vi "Error Handler - UI Loop - cRIO Target Monitoring.vi"(8 "error in (no error)":errorcluster caption="错误输入（无错误）", 11 "Message Queue":refnum<queue> caption="消息队列") -> (3 "dup Message Queue":refnum<queue> caption="消息队列副本")   [LabVIEW 2015]
uses:
  Support VIs/Message Queue/Message Cluster.ctl
  Support VIs/Message Queue/Message Queue.lvlib
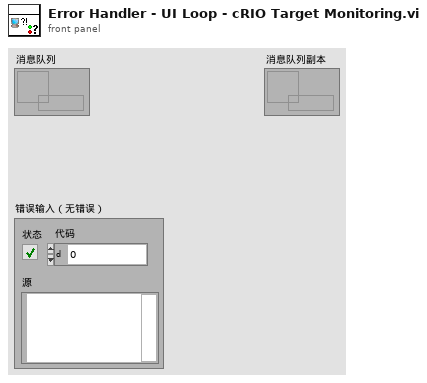
[diagram p1: front panel]
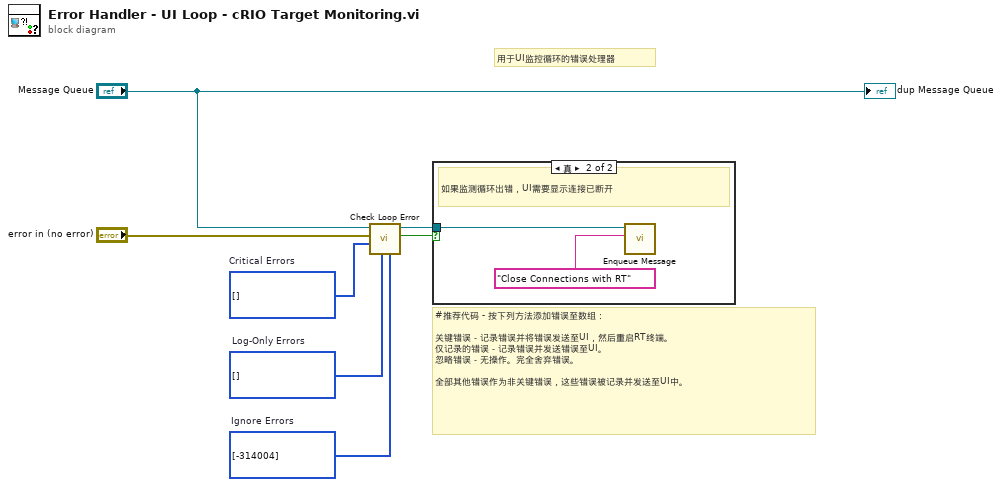
[diagram p0: block diagram]
diagram:
  w5 = i32[] [-314004]  # Ignore Errors
  w6 = i32[] []  # Log-Only Errors
  w7 = i32[] []  # Critical Errors
  # "#推荐代码 - 按下列方法添加错误至数组：\n\n关键错误－记录错误并将错误发送至UI，然后重启RT终端。\n仅记录的错误－记录错误并发送错误至UI。\n忽略错误－无操作。完全舍弃错误。\n\n全部其他错误作为非关键错误，这些错误被记录并发送至UI中。"
  # "用于UI监控循环的错误处理器"
  n1 = call "Check Loop Error.vi"("Ignore Errors"=w5, "Log-Only Errors"=w6, "Critical Errors"=w7, "error to process"="error in (no error)", "Message Queue"="Message Queue") -> ("Enqueued Error?"=w1:bool, "dup Message Queue"=w2:refnum<queue>)  [unwired: 5 in]
  n2 = case shown="真" w1 {
    tunnel: w2 -> [_ w9]
    frame False {
      # "无错误"
    }
    frame True {
      # "如果监测循环出错，UI需要显示连接已断开"
      n3 = call "Enqueue Message.vi"("Message"="Close Connections with RT", "Message Queue"=w9) -> ()  [unwired: 8 in, 2 out]
    }
  }
  "dup Message Queue" <- "Message Queue"
